vi "Write ParsedData.vi"(8 "error in (no error)":errorcluster, 10 "ParsedData":refnum<class "ParsedData.lvclass">, 11 "CommandReceived in":refnum<class "CommandReceived.lvclass">) -> (0 "error out":errorcluster, 3 "CommandReceived out":refnum<class "CommandReceived.lvclass">)   [LabVIEW 2022 SP3, in "Cli.lvlib" / "CommandReceived.lvclass"]
uses:
  CommandReceived.lvclass
  CommandReceived.lvclass/CommandReceived.ctl
  ArgumentParser/Source/ParsedData/ParsedData.lvclass
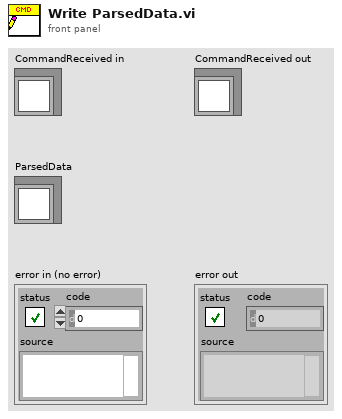
[diagram p1: front panel]
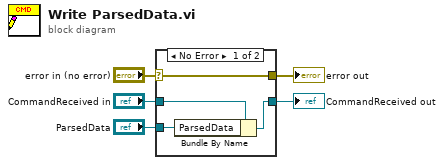
[diagram p0: block diagram]
diagram:
  n1 = case shown="No Error" "error in (no error)" {
    selector: "error in (no error)" -> [w9 w10]
    tunnel: [w9 w10] -> w4
    tunnel: [w7 w11] -> w2
    tunnel: "CommandReceived in" -> [w8 w11]
    tunnel: "ParsedData" -> [w6 _]
    frame No Error {
      n2 = Bundle By Name(cluster=w8, "ParsedData"=w6) -> (w7:refnum<class "CommandReceived.lvclass">)
    }
    frame Error {
    }
  }
  "error out" <- w4
  "CommandReceived out" <- w2
